vi "Load from Type.vi"(8 "error in (no error)":errorcluster, 10 "Control Reference":refnum<vi>) -> (0 "error out":errorcluster, 3 "Control Info out":refnum<class "Control Info.lvclass">)   [LabVIEW 2017, in "Localization.lvlib" / "Control Info.lvclass"]
doc: "Sets the Control Reference to the class data and uses that control reference to determine the class to load and then loads the class.\n\nChoose Movement Consulting, LLC"
uses:
  Control Info.lvclass
  Control Info.lvclass/Control Info.ctl
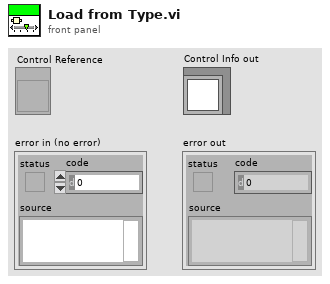
[diagram p1: front panel]
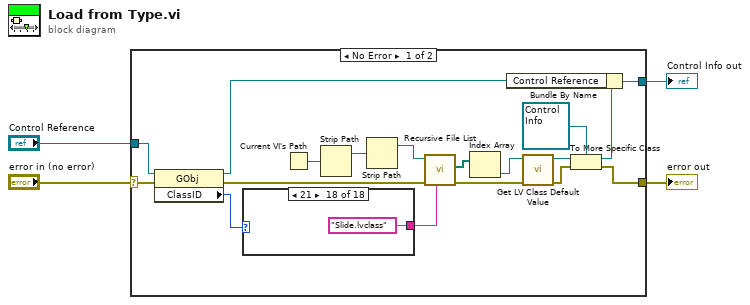
[diagram p0: block diagram]
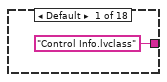
[diagram p2: hidden frame]
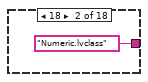
[diagram p3: hidden frame]
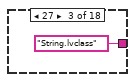
[diagram p4: hidden frame]
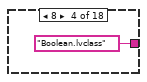
[diagram p5: hidden frame]
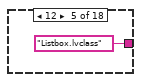
[diagram p6: hidden frame]
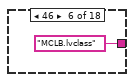
[diagram p7: hidden frame]
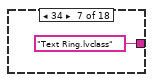
[diagram p8: hidden frame]
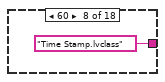
[diagram p9: hidden frame]
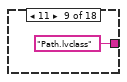
[diagram p10: hidden frame]
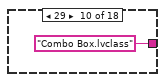
[diagram p11: hidden frame]
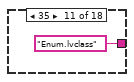
[diagram p12: hidden frame]
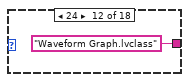
[diagram p13: hidden frame]
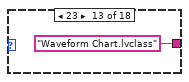
[diagram p14: hidden frame]
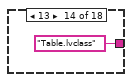
[diagram p15: hidden frame]
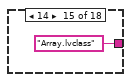
[diagram p16: hidden frame]
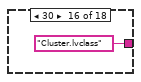
[diagram p17: hidden frame]
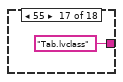
[diagram p18: hidden frame]
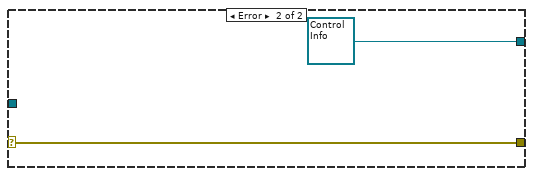
[diagram p19: hidden frame]
diagram:
  n1 = case shown="No Error" "error in (no error)" {
    selector: "error in (no error)" -> [w19 w42]
    tunnel: [w5 w42] -> w3
    tunnel: [w22 refnum<class "Control Info.lvclass"> refnum ("Control Info.lvclass")] -> w1
    tunnel: "Control Reference" -> [w21 _]
    frame No Error {
      n2 = property class="GObj"(reference=w21, error in=w19) -> (reference out=w20:refnum<vi>, error out=w17:errorcluster, "ClassID"=w18:u32)
      n3 = case shown="21" w18 {
        tunnel: ["Control Info.lvclass" "Numeric.lvclass" "String.lvclass" "Boolean.lvclass" "Listbox.lvclass" "MCLB.lvclass" "Text Ring.lvclass" "Time Stamp.lvclass" "Path.lvclass" "Combo Box.lvclass" "Enum.lvclass" "Waveform Graph.lvclass" "Waveform Chart.lvclass" "Table.lvclass" "Array.lvclass" "Cluster.lvclass" "Tab.lvclass" "Slide.lvclass"] -> w12
        frame Default {
        }
        frame 18 {
        }
        frame 27 {
        }
        frame 8 {
        }
        frame 12 {
        }
        frame 46 {
        }
        frame 34 {
        }
        frame 60 {
        }
        frame 11 {
        }
        frame 29 {
        }
        frame 35 {
        }
        frame 24 {
        }
        frame 23 {
        }
        frame 13 {
        }
        frame 14 {
        }
        frame 30 {
        }
        frame 55 {
        }
        frame 21 {
        }
      }
      n4 = Current VI's Path() -> (path=w15:path)
      n5 = Strip Path(path=w15) -> (stripped path=w14:path)  [unwired: 1 out]
      n6 = Strip Path(path=w14) -> (stripped path=w13:path)  [unwired: 1 out]
      n7 = call <vilib>:"Recursive File List.vi"("pattern"=w12, "error in (no error)"=w17, "Folder Path"=w13) -> ("error out"=w16:errorcluster, "All Files in Dir"=w11:path[])  [unwired: 4 in, 3 out]
      n8 = Index Array(array=w11) -> (element=w10:path)  [unwired: 1 in]
      n9 = call <vilib>:"Get LV Class Default Value.vi"("error in (no error)"=w16, "class path"=w10) -> ("error out"=w6:errorcluster, "object"=w9:refnum<class>)  [unwired: 8 in]
      n10 = To More Specific Class(target class=refnum<class "Control Info.lvclass"> refnum ("Control Info.lvclass"), reference=w9, error in=w6) -> (specific class reference=w7:refnum<class "Control Info.lvclass">, error out=w5:errorcluster)
      n11 = Bundle By Name(cluster=w7, "Control Reference"=w20) -> (w22:refnum<class "Control Info.lvclass">)
    }
    frame Error {
    }
  }
  "error out" <- w3
  "Control Info out" <- w1
